vi "ReverseDrive.vi"(7 "cReverseDrive":bool, 9 "Right":dbl, 10 "Left":dbl) -> (1 "Right":dbl, 2 "Left":dbl)   [LabVIEW 2013]
doc: "Reverses driving, back is driven as front would be in a forward drive."
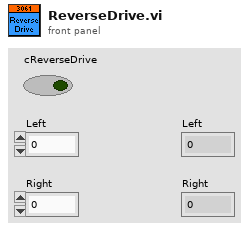
[diagram p1: front panel]
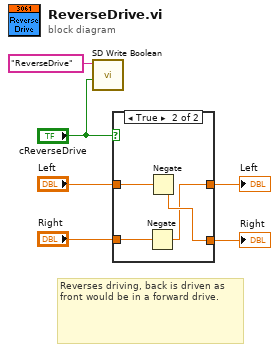
[diagram p0: block diagram]
diagram:
  # "Reverses driving, back is driven as front would be in a forward drive."
  n1 = call <vilib>:"SD Write Boolean.vi"("Boolean"="cReverseDrive", "Name"="ReverseDrive") -> ()  [unwired: 8 in, 2 out]
  n2 = case shown="True" "cReverseDrive" {
    tunnel: [w8 w9] -> w5
    tunnel: "Left" -> [w8 w11]
    tunnel: [w7 w10] -> w3
    tunnel: "Right" -> [w7 w12]
    frame False {
    }
    frame True {
      n3 = Negate(x=w12) -> (-x=w9:dbl)
      n4 = Negate(x=w11) -> (-x=w10:dbl)
    }
  }
  "Left" <- w5
  "Right" <- w3
